vi "Arm.vi"(11 "input cluster":T1) -> ()   [LabVIEW 2015]
uses:
  Joystick/ControlsToCommands.ctl
  References/Refnums.vi
panel:
  out "Bottom Limit Actually Top":bool
  out "Top Limit Actually Bottom":bool
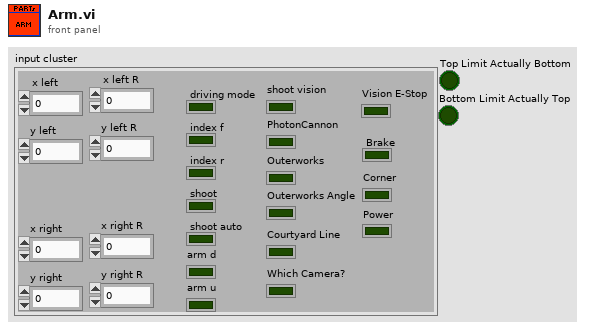
[diagram p1: front panel]
types:
  T1 = typedef "ControlsToCommands.ctl" = cluster{"x left":dbl, "y left":dbl, "x right":dbl, "y right":dbl, "driving mode":bool, "index f":bool, "index r":bool, "shoot":bool, "shoot auto":bool, "arm d":bool, "arm u":bool, "shoot vision":bool, "PhotonCannon":bool, "Outerworks":bool, "Outerworks Angle":bool, "Courtyard Line":bool, "Which Camera?":bool, "Vision E-Stop":bool, "x left R":dbl, "y left R":dbl, "x right R":dbl, "y right R":dbl, "Brake":bool, "Corner":bool, "Power":bool}
  T2 = typedef "WPI_MotorControlDeviceRef.ctl" = cluster{"DeviceStatus":errorcluster, "Type":T3, "PWM":cluster{"PWM Channel":T4, "DeadBand":T5}, "CAN":cluster{"Device Number":u8, "Control Mode":T6, "Semaphore":T7, "Max Vout":dbl, "TalonSRX Control Mode":T8}, "Invert":bool}
  T3 = typedef "WPI_MotorControlType.ctl" = enum16{"PWM", "CAN", "CANTalonSRX"}
  T4 = typedef "FPGA_DIOPWMChannel.ctl" = enum8{"PWM 0", "PWM 1", "PWM 2", "PWM 3", "PWM 4", "PWM 5", "PWM 6", "PWM 7", "PWM 8", "PWM 9", "PWM MXP 0", "PWM MXP 1", "PWM MXP 2", "PWM MXP 3", "PWM MXP 4", "PWM MXP 5", "PWM MXP 6", "PWM MXP 7", "PWM MXP 8", "PWM MXP 9", "Invalid"}
  T5 = typedef "WPI_PWMDeadband.ctl" = cluster{"Name":string, "maxPositivePwm":i32, "minPositivePwm":i32, "centerPwm":i32, "maxNegativePwm":i32, "minNegativePwm":i32, "angularRange":u16}
  T6 = typedef "WPI_CANJaguar_ControlMode.ctl" = enum8{"Percent VBus", "Current", "Speed", "Position", "Voltage"}
  T7 = typedef "Semaphore RefNum" = refnum<k1>
  T8 = typedef "WPI_CANTalonSRX_APIControlMode.ctl" = enum8{"Percent VBus", "Speed", "Position", "Slave", "Unchanged / Invalid", "Voltage Compensation", "Current", "Motion Profile"}
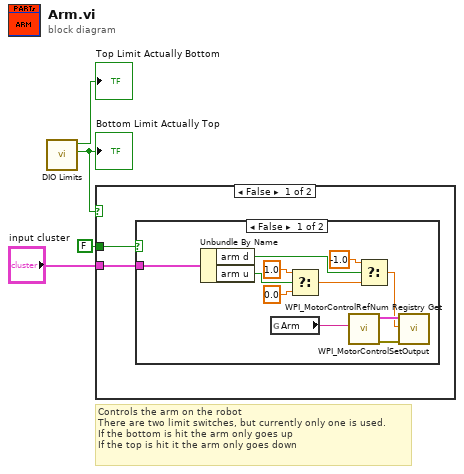
[diagram p0: block diagram]
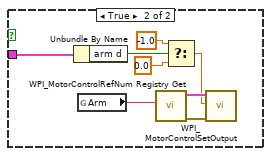
[diagram p2: hidden frame]
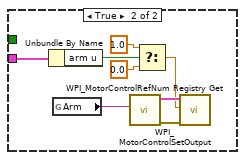
[diagram p3: hidden frame]
diagram:
  # "Controls the arm on the robot\nThere are two limit switches, but currently only one is used.\nIf the bottom is hit the arm only goes up\nIf the top is hit it the arm only goes down"
  n1 = call "DIO Limits.vi"() -> ("Bottom Limit"=w2:bool, "Top Limit"=→"Top Limit Actually Bottom":bool)  [unwired: 10 in]
  "Bottom Limit Actually Top" <- w2
  n2 = case shown="False" w2 {
    tunnel: "input cluster" -> [w6 w27]
    tunnel: FALSE ("Top Limit") -> [w5 _]
    frame False {
      n3 = case shown="False" w5 {
        tunnel: w6 -> [w10 w21]
        frame False {
          n4 = Unbundle By Name(w10) -> ("arm d"=w8:bool, "arm u"=w9:bool)
          n5 = global read "Refnums.vi" "Arm"() -> (w17:string)
          n6 = Select(t=1.0, s=w9, f=0.0) -> (s? t:f=w12:dbl)
          n7 = call <vilib>:"WPI_MotorControlRefNum Registry Get.vi"("refnum name"=w17) -> ("error out"=w11:errorcluster, "MotorControlDevRef"=w16:T2)  [unwired: 9 in]
          n8 = Select(t=-1.0, s=w8, f=w12) -> (s? t:f=w7:dbl)
          n9 = call <vilib>:"WPI_MotorControlSetOutput.vi"("error in (no error)"=w11, "Output"=w7, "MotorControlDevRef"=w16) -> ()  [unwired: 6 in, 3 out]
        }
        frame True {
          n10 = Unbundle By Name(w21) -> ("arm d"=w19:bool)
          n11 = global read "Refnums.vi" "Arm"() -> (w25:string)
          n12 = call <vilib>:"WPI_MotorControlRefNum Registry Get.vi"("refnum name"=w25) -> ("error out"=w22:errorcluster, "MotorControlDevRef"=w24:T2)  [unwired: 9 in]
          n13 = Select(t=-1.0, s=w19, f=0.0) -> (s? t:f=w18:dbl)
          n14 = call <vilib>:"WPI_MotorControlSetOutput.vi"("error in (no error)"=w22, "Output"=w18, "MotorControlDevRef"=w24) -> ()  [unwired: 6 in, 3 out]
        }
      }
    }
    frame True {
      n15 = Unbundle By Name(w27) -> ("arm u"=w31:bool)
      n16 = global read "Refnums.vi" "Arm"() -> (w33:string)
      n17 = call <vilib>:"WPI_MotorControlRefNum Registry Get.vi"("refnum name"=w33) -> ("error out"=w28:errorcluster, "MotorControlDevRef"=w32:T2)  [unwired: 9 in]
      n18 = Select(t=1.0, s=w31, f=0.0) -> (s? t:f=w26:dbl)
      n19 = call <vilib>:"WPI_MotorControlSetOutput.vi"("error in (no error)"=w28, "Output"=w26, "MotorControlDevRef"=w32) -> ()  [unwired: 6 in, 3 out]
    }
  }
